vi "PathPlanner_PathFinder_Key.vi"(6 "eps_little":dbl, 8 "Sstart":T1, 9 "G":map{i32, dbl}(c390), 10 "RHS":map{i32, dbl}(c390), 11 "S":T1) -> (3 "DoublePair":T2)   [LabVIEW 2019]
uses:
  PathPlannerLib24/TypeDef/PathPlannerFinderGridPosition.ctl
  PathPlannerLib24/TypeDef/PathPlannerFinderDoublePair.ctl
  PathPlannerLib24/VI/PathPlanner_GridPosition_Get.vi
  PathPlannerLib24/PathPlanner24.lvlib
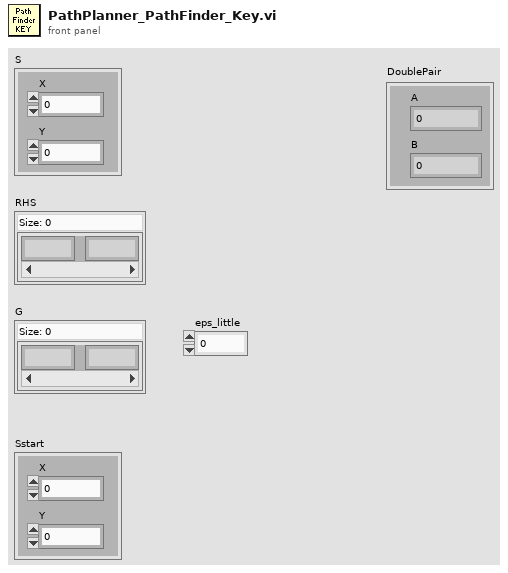
[diagram p1: front panel]
types:
  T1 = typedef "PathPlanner24.lvlib/PathPlannerFinderGridPosition.ctl" = cluster{"X":i32, "Y":i32}
  T2 = typedef "PathPlanner24.lvlib/PathPlannerFinderDoublePair.ctl" = cluster{"A":dbl, "B":dbl}
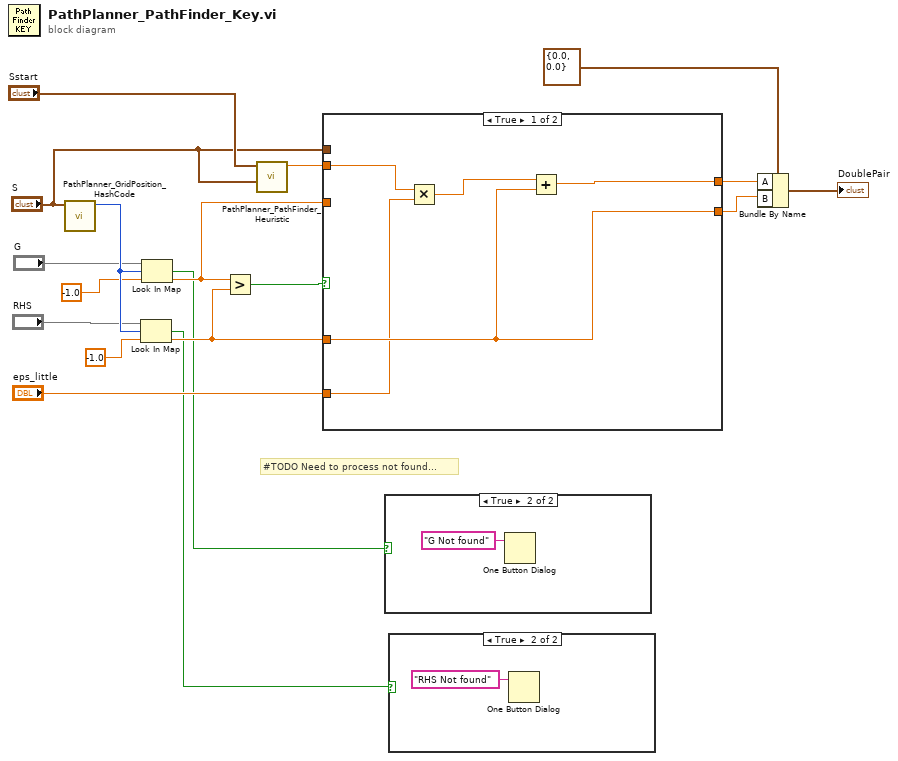
[diagram p0: block diagram]
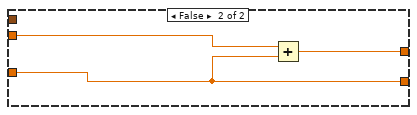
[diagram p4: hidden frame]
diagram:
  # "#TODO Need to process not found..."
  n1 = call "PathPlanner_GridPosition_HashCode.vi"("GridPosition"="S") -> ("HashCode"=w18:i32)  [unwired: 10 in]
  n2 = Look In Map(map="RHS", key=w18, default value=-1.0) -> (key not found?=w1:bool, value=w9:dbl)
  n3 = Look In Map(map="G", key=w18, default value=-1.0) -> (key not found?=w2:bool, value=w14:dbl)
  n4 = Greater?(x=w14, y=w9) -> (0:w15:bool)
  n5 = call "PathPlanner_PathFinder_Heuristic.vi"("sGoalLoc"="S", "sStartLoc"="Sstart") -> ("heuristic"=w8:dbl)  [unwired: 9 in]
  n6 = case shown="True" w15 {
    tunnel: w14 -> [_ w24]
    tunnel: [w23 w26] -> w13
    tunnel: [w22 w24] -> w12
    tunnel: w9 -> [w22 _]
    tunnel: "S" -> [_ _]
    tunnel: w8 -> [w21 w25]
    tunnel: "eps_little" -> [w19 _]
    frame True {
      n7 = Multiply(x=w21, y=w19) -> (x*y=w20:dbl)
      n8 = Add(x=w20, y=w22) -> (x+y=w23:dbl)
    }
    frame False {
      n9 = Add(x=w25, y=w24) -> (x+y=w26:dbl)
    }
  }
  n10 = case shown="True" w2 {
    frame False {
    }
    frame True {
      n11 = One Button Dialog(message="G Not found") -> ()  [unwired: 1 in, 1 out]
    }
  }
  n12 = case shown="True" w1 {
    frame False {
    }
    frame True {
      n13 = One Button Dialog(message="RHS Not found") -> ()  [unwired: 1 in, 1 out]
    }
  }
  n14 = Bundle By Name(cluster=T2 {"A"=0.0, "B"=0.0} ("DoublePair"), "A"=w13, "B"=w12) -> (→"DoublePair":T2)
